vi "StateMachine.vi"() -> ()   [LabVIEW 2015]
panel:
  out "String":string="Estado Inicial"
  out "Enum":T1(ring)
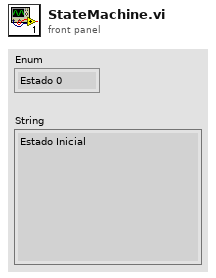
[diagram p1: front panel]
types:
  T1 = enum16{"Estado 0", "Estado 1", "Estado 2", "Estado 3", "Estado 4"}
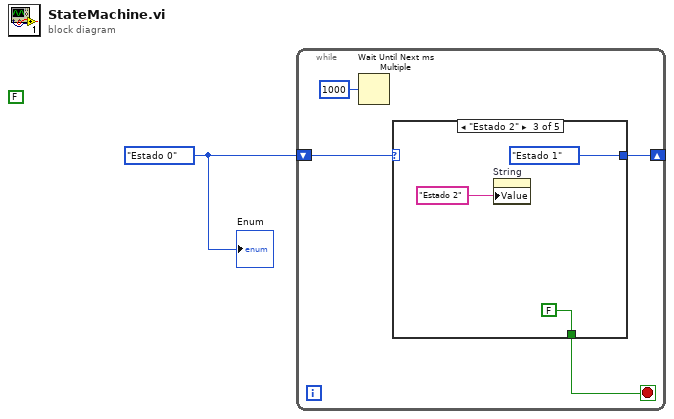
[diagram p0: block diagram]
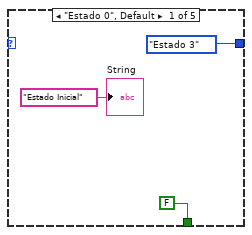
[diagram p2: hidden frame]
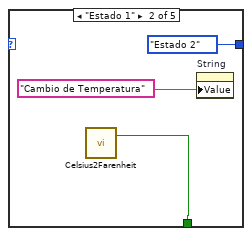
[diagram p3: hidden frame]
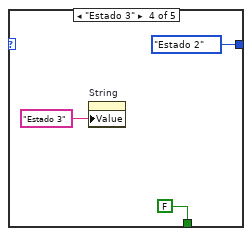
[diagram p4: hidden frame]
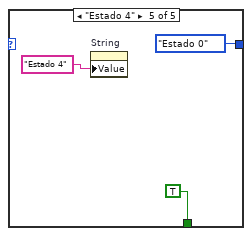
[diagram p5: hidden frame]
diagram:
  (unwired) FALSE
  w1 = T1."Estado 0"
  n1 = while {
    shift-right: [w3] -> _
    shift-left: w1 -> [w4]
    stop <- w2 stop-if-true
    n2 = Wait Until Next ms Multiple(millisecond multiple=u32 1000) -> ()  [unwired: 1 out]
    n3 = case shown="\"Estado 2\"" w4 {
      tunnel: [T1."Estado 3" T1."Estado 2" T1."Estado 1" T1."Estado 2" T1."Estado 0"] -> w3
      tunnel: [FALSE ("stop") w9 FALSE ("stop") FALSE ("stop") TRUE ("stop")] -> w2
      frame "Estado 0", Default {
        "String" <- "Estado Inicial"
      }
      frame "Estado 1" {
        n4 = call "Celsius2Farenheit.vi"() -> ("stop 2"=w9:bool)  [unwired: 1 in, 1 out]
        n5 = property on="String" class="Str"("Value"="Cambio de Temperatura") -> ()  [unwired: 2 in, 2 out]
      }
      frame "Estado 2" {
        n6 = property on="String" class="Str"("Value"="Estado 2") -> ()  [unwired: 2 in, 2 out]
      }
      frame "Estado 3" {
        n7 = property on="String" class="Str"("Value"="Estado 3") -> ()  [unwired: 2 in, 2 out]
      }
      frame "Estado 4" {
        n8 = property on="String" class="Str"("Value"="Estado 4") -> ()  [unwired: 2 in, 2 out]
      }
    }
  }
  "Enum" <- w1
